vi "MR_Build-A-Block.vi"(1 "Build-A-Block":T2(array[cluster])=[{"Row Type Selector"=enum."Wait (minutes)", "Index"=0.0, "Direction"=enum."Forward"}, {"Row Type Selector"=enum."Vertical Profile", "Index"=0.0, "Direction"=enum."Forward"}, {"Row Type Selector"=enum."Vertical Profile", "Index"=1.0, "Direction"=enum."Forward"}, {"Row Type Selector"=enum."Move Traverse Only", "Index"=0.0, "Direction"=enum."Forward"}, {"Row Type Selector"=enum."Send Message", "Index"=0.0, "Direction"=enum."Forward"}, {"Row Type Selector"=enum."Blank Row", "Index"=0.0, "Direction"=enum."Forward"}]) -> (0 "TaskArray":T5(array[cluster])=[{"Start X"=-3390.0, "Start Y"=-113.0, "Start Z"=780.0, "End X"=-3390.0, "End Y"=-113.0, "End Z"=780.0, "No. of pts."=0, "Spacing"=enum."Linear", "Filename"=path "", "Tunnel Speed"=7.64, "Averaging time (min)"=0.0, "Extra Commands"="", "Carrier_1 Q (l/min)"=0.0, "Carrier_2 Q (l/min)"=0.0, "Trace Gas Concentration (%)"=0.0, "Specific Arguments"="", "Comments"="Tunnel Warm Up", "Row No"=0, "Row Type Selector"=enum."Set Tunnel Speed Only", "Completion time"="", "Row Duration (mins)"=10.0, "No. of Valid pts."=0, "Meas Setup File"=""}, {"Start X"=-3390.0, "Start Y"=-113.0, "Start Z"=780.0, "End X"=-3390.0, "End Y"=-113.0, "End Z"=780.0, "No. of pts."=0, "Spacing"=enum."Linear", "Filename"=path "", "Tunnel Speed"=7.64, "Averaging time (min)"=0.0, "Extra Commands"="", "Carrier_1 Q (l/min)"=0.0, "Carrier_2 Q (l/min)"=0.0, "Trace Gas Concentration (%)"=0.0, "Specific Arguments"="10", "Comments"="Tunnel Warm Up", "Row No"=0, "Row Type Selector"=enum."Wait (minutes)", "Completion time"="", "Row Duration (mins)"=0.0, "No. of Valid pts."=0, "Meas Setup File"=""}, {"Start X"=0.0, "Start Y"=0.0, "Start Z"=150.0, "End X"=0.0, "End Y"=0.0, "End Z"=150.0, "No. of pts."=0, "Spacing"=enum."Linear", "Filename"=path "", "Tunnel Speed"=7.64, "Averaging time (min)"=0.0, "Extra Commands"="!Work in Tunnel Coordinates", "Carrier_1 Q (l/min)"=0.0, "Carrier_2 Q (l/min)"=0.0, "Trace Gas Concentration (%)"=0.0, "Specific Arguments"="", "Comments"="", "Row No"=0, "Row Type Selector"=enum."Move Traverse Only", "Completion time"="", "Row Duration (mins)"=0.0, "No. of Valid pts."=0, "Meas Setup File"=""}, {"Start X"=0.0, "Start Y"=0.0, "Start Z"=805.0, "End X"=0.0, "End Y"=0.0, "End Z"=805.0, "No. of pts."=0, "Spacing"=enum."Linear", "Filename"=path "", "Tunnel Speed"=7.64, "Averaging time (min)"=0.0, "Extra Commands"="!Work in Tunnel Coordinates", "Carrier_1 Q (l/min)"=0.0, "Carrier_2 Q (l/min)"=0.0, "Trace Gas Concentration (%)"=0.0, "Specific Arguments"="MoveTT.vi;10", "Comments"="", "Row No"=0, "Row Type Selector"=enum."Run VI Named:", "Completion time"="", "Row Duration (mins)"=0.0, "No. of Valid pts."=0, "Meas Setup File"=""}, {"Start X"=-72.9, "Start Y"=-56.5, "Start Z"=12.7, "End X"=-72.9, "End Y"=-56.5, "End Z"=25.4, "No. of pts."=3, "Spacing"=enum."Specified", "Filename"=path "M:/\\Projects\\8773\\Results\\Tunnel1\\AnemometerSurvey.xls", "Tunnel Speed"=7.64, "Averaging time (min)"=1.0, "Extra Commands"="", "Carrier_1 Q (l/min)"=0.0, "Carrier_2 Q (l/min)"=0.0, "Trace Gas Concentration (%)"=0.0, "Specific Arguments"="Z= ;12.7;19.1;25.4\r", "Comments"="Anemo1", "Row No"=0, "Row Type Selector"=enum."Vertical Profile", "Completion time"="", "Row Duration (mins)"=0.0, "No. of Valid pts."=0, "Meas Setup File"="Current_Setup.xls"}, {"Start X"=-458.4, "Start Y"=87.9, "Start Z"=25.6, "End X"=-458.4, "End Y"=87.9, "End Z"=38.3, "No. of pts."=3, "Spacing"=enum."Specified", "Filename"=path "M:/\\Projects\\8773\\Results\\Tunnel1\\AnemometerSurvey.xls", "Tunnel Speed"=7.64, "Averaging time (min)"=1.0, "Extra Commands"="", "Carrier_1 Q (l/min)"=0.0, "Carrier_2 Q (l/min)"=0.0, "Trace Gas Concentration (%)"=0.0, "Specific Arguments"="Z= ;25.6;32.0;38.3\r", "Comments"="Anemo2", "Row No"=0, "Row Type Selector"=enum."Vertical Profile", "Completion time"="", "Row Duration (mins)"=0.0, "No. of Valid pts."=0, "Meas Setup File"="Current_Setup.xls"}, {"Start X"=0.0, "Start Y"=0.0, "Start Z"=150.0, "End X"=0.0, "End Y"=0.0, "End Z"=150.0, "No. of pts."=0, "Spacing"=enum."Linear", "Filename"=path "", "Tunnel Speed"=7.64, "Averaging time (min)"=0.0, "Extra Commands"="!Work in Tunnel Coordinates", "Carrier_1 Q (l/min)"=0.0, "Carrier_2 Q (l/min)"=0.0, "Trace Gas Concentration (%)"=0.0, "Specific Arguments"="", "Comments"="", "Row No"=0, "Row Type Selector"=enum."Move Traverse Only", "Completion time"="", "Row Duration (mins)"=0.0, "No. of Valid pts."=0, "Meas Setup File"=""}, {"Start X"=0.0, "Start Y"=0.0, "Start Z"=805.0, "End X"=0.0, "End Y"=0.0, "End Z"=805.0, "No. of pts."=0, "Spacing"=enum."Linear", "Filename"=path "", "Tunnel Speed"=7.64, "Averaging time (min)"=0.0, "Extra Commands"="!Work in Tunnel Coordinates", "Carrier_1 Q (l/min)"=0.0, "Carrier_2 Q (l/min)"=0.0, "Trace Gas Concentration (%)"=0.0, "Specific Arguments"="MoveTT.vi;30", "Comments"="", "Row No"=0, "Row Type Selector"=enum."Run VI Named:", "Completion time"="", "Row Duration (mins)"=0.0, "No. of Valid pts."=0, "Meas Setup File"=""}, {"Start X"=-72.9, "Start Y"=-56.5, "Start Z"=12.7, "End X"=-72.9, "End Y"=-56.5, "End Z"=25.4, "No. of pts."=3, "Spacing"=enum."Specified", "Filename"=path "M:/\\Projects\\8773\\Results\\Tunnel1\\AnemometerSurvey.xls", "Tunnel Speed"=7.64, "Averaging time (min)"=1.0, "Extra Commands"="", "Carrier_1 Q (l/min)"=0.0, "Carrier_2 Q (l/min)"=0.0, "Trace Gas Concentration (%)"=0.0, "Specific Arguments"="Z= ;12.7;19.1;25.4\r", "Comments"="Anemo1", "Row No"=0, "Row Type Selector"=enum."Vertical Profile", "Completion time"="", "Row Duration (mins)"=0.0, "No. of Valid pts."=0, "Meas Setup File"="Current_Setup.xls"}, {"Start X"=-458.4, "Start Y"=87.9, "Start Z"=25.6, "End X"=-458.4, "End Y"=87.9, "End Z"=38.3, "No. of pts."=3, "Spacing"=enum."Specified", "Filename"=path "M:/\\Projects\\8773\\Results\\Tunnel1\\AnemometerSurvey.xls", "Tunnel Speed"=7.64, "Averaging time (min)"=1.0, "Extra Commands"="", "Carrier_1 Q (l/min)"=0.0, "Carrier_2 Q (l/min)"=0.0, "Trace Gas Concentration (%)"=0.0, "Specific Arguments"="Z= ;25.6;32.0;38.3\r", "Comments"="Anemo2", "Row No"=0, "Row Type Selector"=enum."Vertical Profile", "Completion time"="", "Row Duration (mins)"=0.0, "No. of Valid pts."=0, "Meas Setup File"="Current_Setup.xls"}, {"Start X"=0.0, "Start Y"=0.0, "Start Z"=150.0, "End X"=0.0, "End Y"=0.0, "End Z"=150.0, "No. of pts."=0, "Spacing"=enum."Linear", "Filename"=path "", "Tunnel Speed"=7.64, "Averaging time (min)"=0.0, "Extra Commands"="!Work in Tunnel Coordinates", "Carrier_1 Q (l/min)"=0.0, "Carrier_2 Q (l/min)"=0.0, "Trace Gas Concentration (%)"=0.0, "Specific Arguments"="", "Comments"="", "Row No"=0, "Row Type Selector"=enum."Move Traverse Only", "Completion time"="", "Row Duration (mins)"=0.0, "No. of Valid pts."=0, "Meas Setup File"=""}, {"Start X"=0.0, "Start Y"=0.0, "Start Z"=805.0, "End X"=0.0, "End Y"=0.0, "End Z"=805.0, "No. of pts."=0, "Spacing"=enum."Linear", "Filename"=path "", "Tunnel Speed"=7.64, "Averaging time (min)"=0.0, "Extra Commands"="!Work in Tunnel Coordinates", "Carrier_1 Q (l/min)"=0.0, "Carrier_2 Q (l/min)"=0.0, "Trace Gas Concentration (%)"=0.0, "Specific Arguments"="MoveTT.vi;50", "Comments"="", "Row No"=0, "Row Type Selector"=enum."Run VI Named:", "Completion time"="", "Row Duration (mins)"=0.0, "No. of Valid pts."=0, "Meas Setup File"=""}, {"Start X"=-72.9, "Start Y"=-56.5, "Start Z"=12.7, "End X"=-72.9, "End Y"=-56.5, "End Z"=25.4, "No. of pts."=3, "Spacing"=enum."Specified", "Filename"=path "M:/\\Projects\\8773\\Results\\Tunnel1\\AnemometerSurvey.xls", "Tunnel Speed"=7.64, "Averaging time (min)"=1.0, "Extra Commands"="", "Carrier_1 Q (l/min)"=0.0, "Carrier_2 Q (l/min)"=0.0, "Trace Gas Concentration (%)"=0.0, "Specific Arguments"="Z= ;12.7;19.1;25.4\r", "Comments"="Anemo1", "Row No"=0, "Row Type Selector"=enum."Vertical Profile", "Completion time"="", "Row Duration (mins)"=0.0, "No. of Valid pts."=0, "Meas Setup File"="Current_Setup.xls"}, {"Start X"=-458.4, "Start Y"=87.9, "Start Z"=25.6, "End X"=-458.4, "End Y"=87.9, "End Z"=38.3, "No. of pts."=3, "Spacing"=enum."Specified", "Filename"=path "M:/\\Projects\\8773\\Results\\Tunnel1\\AnemometerSurvey.xls", "Tunnel Speed"=7.64, "Averaging time (min)"=1.0, "Extra Commands"="", "Carrier_1 Q (l/min)"=0.0, "Carrier_2 Q (l/min)"=0.0, "Trace Gas Concentration (%)"=0.0, "Specific Arguments"="Z= ;25.6;32.0;38.3\r", "Comments"="Anemo2", "Row No"=0, "Row Type Selector"=enum."Vertical Profile", "Completion time"="", "Row Duration (mins)"=0.0, "No. of Valid pts."=0, "Meas Setup File"="Current_Setup.xls"}, {"Start X"=0.0, "Start Y"=0.0, "Start Z"=150.0, "End X"=0.0, "End Y"=0.0, "End Z"=150.0, "No. of pts."=0, "Spacing"=enum."Linear", "Filename"=path "", "Tunnel Speed"=7.64, "Averaging time (min)"=0.0, "Extra Commands"="!Work in Tunnel Coordinates", "Carrier_1 Q (l/min)"=0.0, "Carrier_2 Q (l/min)"=0.0, "Trace Gas Concentration (%)"=0.0, "Specific Arguments"="", "Comments"="", "Row No"=0, "Row Type Selector"=enum."Move Traverse Only", "Completion time"="", "Row Duration (mins)"=0.0, "No. of Valid pts."=0, "Meas Setup File"=""}, {"Start X"=0.0, "Start Y"=0.0, "Start Z"=805.0, "End X"=0.0, "End Y"=0.0, "End Z"=805.0, "No. of pts."=0, "Spacing"=enum."Linear", "Filename"=path "", "Tunnel Speed"=7.64, "Averaging time (min)"=0.0, "Extra Commands"="!Work in Tunnel Coordinates", "Carrier_1 Q (l/min)"=0.0, "Carrier_2 Q (l/min)"=0.0, "Trace Gas Concentration (%)"=0.0, "Specific Arguments"="MoveTT.vi;70", "Comments"="", "Row No"=0, "Row Type Selector"=enum."Run VI Named:", "Completion time"="", "Row Duration (mins)"=0.0, "No. of Valid pts."=0, "Meas Setup File"=""}, {"Start X"=-72.9, "Start Y"=-56.5, "Start Z"=12.7, "End X"=-72.9, "End Y"=-56.5, "End Z"=25.4, "No. of pts."=3, "Spacing"=enum."Specified", "Filename"=path "M:/\\Projects\\8773\\Results\\Tunnel1\\AnemometerSurvey.xls", "Tunnel Speed"=7.64, "Averaging time (min)"=1.0, "Extra Commands"="", "Carrier_1 Q (l/min)"=0.0, "Carrier_2 Q (l/min)"=0.0, "Trace Gas Concentration (%)"=0.0, "Specific Arguments"="Z= ;12.7;19.1;25.4\r", "Comments"="Anemo1", "Row No"=0, "Row Type Selector"=enum."Vertical Profile", "Completion time"="", "Row Duration (mins)"=0.0, "No. of Valid pts."=0, "Meas Setup File"="Current_Setup.xls"}, {"Start X"=-458.4, "Start Y"=87.9, "Start Z"=25.6, "End X"=-458.4, "End Y"=87.9, "End Z"=38.3, "No. of pts."=3, "Spacing"=enum."Specified", "Filename"=path "M:/\\Projects\\8773\\Results\\Tunnel1\\AnemometerSurvey.xls", "Tunnel Speed"=7.64, "Averaging time (min)"=1.0, "Extra Commands"="", "Carrier_1 Q (l/min)"=0.0, "Carrier_2 Q (l/min)"=0.0, "Trace Gas Concentration (%)"=0.0, "Specific Arguments"="Z= ;25.6;32.0;38.3\r", "Comments"="Anemo2", "Row No"=0, "Row Type Selector"=enum."Vertical Profile", "Completion time"="", "Row Duration (mins)"=0.0, "No. of Valid pts."=0, "Meas Setup File"="Current_Setup.xls"}, {"Start X"=0.0, "Start Y"=0.0, "Start Z"=150.0, "End X"=0.0, "End Y"=0.0, "End Z"=150.0, "No. of pts."=0, "Spacing"=enum."Linear", "Filename"=path "", "Tunnel Speed"=7.64, "Averaging time (min)"=0.0, "Extra Commands"="!Work in Tunnel Coordinates", "Carrier_1 Q (l/min)"=0.0, "Carrier_2 Q (l/min)"=0.0, "Trace Gas Concentration (%)"=0.0, "Specific Arguments"="", "Comments"="", "Row No"=0, "Row Type Selector"=enum."Move Traverse Only", "Completion time"="", "Row Duration (mins)"=0.0, "No. of Valid pts."=0, "Meas Setup File"=""}, {"Start X"=0.0, "Start Y"=0.0, "Start Z"=805.0, "End X"=0.0, "End Y"=0.0, "End Z"=805.0, "No. of pts."=0, "Spacing"=enum."Linear", "Filename"=path "", "Tunnel Speed"=7.64, "Averaging time (min)"=0.0, "Extra Commands"="!Work in Tunnel Coordinates", "Carrier_1 Q (l/min)"=0.0, "Carrier_2 Q (l/min)"=0.0, "Trace Gas Concentration (%)"=0.0, "Specific Arguments"="MoveTT.vi;90", "Comments"="", "Row No"=0, "Row Type Selector"=enum."Run VI Named:", "Completion time"="", "Row Duration (mins)"=0.0, "No. of Valid pts."=0, "Meas Setup File"=""}, {"Start X"=-72.9, "Start Y"=-56.5, "Start Z"=12.7, "End X"=-72.9, "End Y"=-56.5, "End Z"=25.4, "No. of pts."=3, "Spacing"=enum."Specified", "Filename"=path "M:/\\Projects\\8773\\Results\\Tunnel1\\AnemometerSurvey.xls", "Tunnel Speed"=7.64, "Averaging time (min)"=1.0, "Extra Commands"="", "Carrier_1 Q (l/min)"=0.0, "Carrier_2 Q (l/min)"=0.0, "Trace Gas Concentration (%)"=0.0, "Specific Arguments"="Z= ;12.7;19.1;25.4\r", "Comments"="Anemo1", "Row No"=0, "Row Type Selector"=enum."Vertical Profile", "Completion time"="", "Row Duration (mins)"=0.0, "No. of Valid pts."=0, "Meas Setup File"="Current_Setup.xls"}, {"Start X"=-458.4, "Start Y"=87.9, "Start Z"=25.6, "End X"=-458.4, "End Y"=87.9, "End Z"=38.3, "No. of pts."=3, "Spacing"=enum."Specified", "Filename"=path "M:/\\Projects\\8773\\Results\\Tunnel1\\AnemometerSurvey.xls", "Tunnel Speed"=7.64, "Averaging time (min)"=1.0, "Extra Commands"="", "Carrier_1 Q (l/min)"=0.0, "Carrier_2 Q (l/min)"=0.0, "Trace Gas Concentration (%)"=0.0, "Specific Arguments"="Z= ;25.6;32.0;38.3\r", "Comments"="Anemo2", "Row No"=0, "Row Type Selector"=enum."Vertical Profile", "Completion time"="", "Row Duration (mins)"=0.0, "No. of Valid pts."=0, "Meas Setup File"="Current_Setup.xls"}, {"Start X"=0.0, "Start Y"=0.0, "Start Z"=150.0, "End X"=0.0, "End Y"=0.0, "End Z"=150.0, "No. of pts."=0, "Spacing"=enum."Linear", "Filename"=path "", "Tunnel Speed"=7.64, "Averaging time (min)"=0.0, "Extra Commands"="!Work in Tunnel Coordinates", "Carrier_1 Q (l/min)"=0.0, "Carrier_2 Q (l/min)"=0.0, "Trace Gas Concentration (%)"=0.0, "Specific Arguments"="", "Comments"="", "Row No"=0, "Row Type Selector"=enum."Move Traverse Only", "Completion time"="", "Row Duration (mins)"=0.0, "No. of Valid pts."=0, "Meas Setup File"=""}, {"Start X"=0.0, "Start Y"=0.0, "Start Z"=805.0, "End X"=0.0, "End Y"=0.0, "End Z"=805.0, "No. of pts."=0, "Spacing"=enum."Linear", "Filename"=path "", "Tunnel Speed"=7.64, "Averaging time (min)"=0.0, "Extra Commands"="!Work in Tunnel Coordinates", "Carrier_1 Q (l/min)"=0.0, "Carrier_2 Q (l/min)"=0.0, "Trace Gas Concentration (%)"=0.0, "Specific Arguments"="MoveTT.vi;110", "Comments"="", "Row No"=0, "Row Type Selector"=enum."Run VI Named:", "Completion time"="", "Row Duration (mins)"=0.0, "No. of Valid pts."=0, "Meas Setup File"=""}, {"Start X"=-72.9, "Start Y"=-56.5, "Start Z"=12.7, "End X"=-72.9, "End Y"=-56.5, "End Z"=25.4, "No. of pts."=3, "Spacing"=enum."Specified", "Filename"=path "M:/\\Projects\\8773\\Results\\Tunnel1\\AnemometerSurvey.xls", "Tunnel Speed"=7.64, "Averaging time (min)"=1.0, "Extra Commands"="", "Carrier_1 Q (l/min)"=0.0, "Carrier_2 Q (l/min)"=0.0, "Trace Gas Concentration (%)"=0.0, "Specific Arguments"="Z= ;12.7;19.1;25.4\r", "Comments"="Anemo1", "Row No"=0, "Row Type Selector"=enum."Vertical Profile", "Completion time"="", "Row Duration (mins)"=0.0, "No. of Valid pts."=0, "Meas Setup File"="Current_Setup.xls"}, {"Start X"=-458.4, "Start Y"=87.9, "Start Z"=25.6, "End X"=-458.4, "End Y"=87.9, "End Z"=38.3, "No. of pts."=3, "Spacing"=enum."Specified", "Filename"=path "M:/\\Projects\\8773\\Results\\Tunnel1\\AnemometerSurvey.xls", "Tunnel Speed"=7.64, "Averaging time (min)"=1.0, "Extra Commands"="", "Carrier_1 Q (l/min)"=0.0, "Carrier_2 Q (l/min)"=0.0, "Trace Gas Concentration (%)"=0.0, "Specific Arguments"="Z= ;25.6;32.0;38.3\r", "Comments"="Anemo2", "Row No"=0, "Row Type Selector"=enum."Vertical Profile", "Completion time"="", "Row Duration (mins)"=0.0, "No. of Valid pts."=0, "Meas Setup File"="Current_Setup.xls"}, {"Start X"=0.0, "Start Y"=0.0, "Start Z"=150.0, "End X"=0.0, "End Y"=0.0, "End Z"=150.0, "No. of pts."=0, "Spacing"=enum."Linear", "Filename"=path "", "Tunnel Speed"=7.64, "Averaging time (min)"=0.0, "Extra Commands"="!Work in Tunnel Coordinates", "Carrier_1 Q (l/min)"=0.0, "Carrier_2 Q (l/min)"=0.0, "Trace Gas Concentration (%)"=0.0, "Specific Arguments"="", "Comments"="", "Row No"=0, "Row Type Selector"=enum."Move Traverse Only", "Completion time"="", "Row Duration (mins)"=0.0, "No. of Valid pts."=0, "Meas Setup File"=""}, {"Start X"=0.0, "Start Y"=0.0, "Start Z"=805.0, "End X"=0.0, "End Y"=0.0, "End Z"=805.0, "No. of pts."=0, "Spacing"=enum."Linear", "Filename"=path "", "Tunnel Speed"=7.64, "Averaging time (min)"=0.0, "Extra Commands"="!Work in Tunnel Coordinates", "Carrier_1 Q (l/min)"=0.0, "Carrier_2 Q (l/min)"=0.0, "Trace Gas Concentration (%)"=0.0, "Specific Arguments"="MoveTT.vi;130", "Comments"="", "Row No"=0, "Row Type Selector"=enum."Run VI Named:", "Completion time"="", "Row Duration (mins)"=0.0, "No. of Valid pts."=0, "Meas Setup File"=""}, {"Start X"=-72.9, "Start Y"=-56.5, "Start Z"=12.7, "End X"=-72.9, "End Y"=-56.5, "End Z"=25.4, "No. of pts."=3, "Spacing"=enum."Specified", "Filename"=path "M:/\\Projects\\8773\\Results\\Tunnel1\\AnemometerSurvey.xls", "Tunnel Speed"=7.64, "Averaging time (min)"=1.0, "Extra Commands"="", "Carrier_1 Q (l/min)"=0.0, "Carrier_2 Q (l/min)"=0.0, "Trace Gas Concentration (%)"=0.0, "Specific Arguments"="Z= ;12.7;19.1;25.4\r", "Comments"="Anemo1", "Row No"=0, "Row Type Selector"=enum."Vertical Profile", "Completion time"="", "Row Duration (mins)"=0.0, "No. of Valid pts."=0, "Meas Setup File"="Current_Setup.xls"}, {"Start X"=-458.4, "Start Y"=87.9, "Start Z"=25.6, "End X"=-458.4, "End Y"=87.9, "End Z"=38.3, "No. of pts."=3, "Spacing"=enum."Specified", "Filename"=path "M:/\\Projects\\8773\\Results\\Tunnel1\\AnemometerSurvey.xls", "Tunnel Speed"=7.64, "Averaging time (min)"=1.0, "Extra Commands"="", "Carrier_1 Q (l/min)"=0.0, "Carrier_2 Q (l/min)"=0.0, "Trace Gas Concentration (%)"=0.0, "Specific Arguments"="Z= ;25.6;32.0;38.3\r", "Comments"="Anemo2", "Row No"=0, "Row Type Selector"=enum."Vertical Profile", "Completion time"="", "Row Duration (mins)"=0.0, "No. of Valid pts."=0, "Meas Setup File"="Current_Setup.xls"}, {"Start X"=0.0, "Start Y"=0.0, "Start Z"=150.0, "End X"=0.0, "End Y"=0.0, "End Z"=150.0, "No. of pts."=0, "Spacing"=enum."Linear", "Filename"=path "", "Tunnel Speed"=7.64, "Averaging time (min)"=0.0, "Extra Commands"="!Work in Tunnel Coordinates", "Carrier_1 Q (l/min)"=0.0, "Carrier_2 Q (l/min)"=0.0, "Trace Gas Concentration (%)"=0.0, "Specific Arguments"="", "Comments"="", "Row No"=0, "Row Type Selector"=enum."Move Traverse Only", "Completion time"="", "Row Duration (mins)"=0.0, "No. of Valid pts."=0, "Meas Setup File"=""}, {"Start X"=0.0, "Start Y"=0.0, "Start Z"=805.0, "End X"=0.0, "End Y"=0.0, "End Z"=805.0, "No. of pts."=0, "Spacing"=enum."Linear", "Filename"=path "", "Tunnel Speed"=7.64, "Averaging time (min)"=0.0, "Extra Commands"="!Work in Tunnel Coordinates", "Carrier_1 Q (l/min)"=0.0, "Carrier_2 Q (l/min)"=0.0, "Trace Gas Concentration (%)"=0.0, "Specific Arguments"="MoveTT.vi;150", "Comments"="", "Row No"=0, "Row Type Selector"=enum."Run VI Named:", "Completion time"="", "Row Duration (mins)"=0.0, "No. of Valid pts."=0, "Meas Setup File"=""}, {"Start X"=-72.9, "Start Y"=-56.5, "Start Z"=12.7, "End X"=-72.9, "End Y"=-56.5, "End Z"=25.4, "No. of pts."=3, "Spacing"=enum."Specified", "Filename"=path "M:/\\Projects\\8773\\Results\\Tunnel1\\AnemometerSurvey.xls", "Tunnel Speed"=7.64, "Averaging time (min)"=1.0, "Extra Commands"="", "Carrier_1 Q (l/min)"=0.0, "Carrier_2 Q (l/min)"=0.0, "Trace Gas Concentration (%)"=0.0, "Specific Arguments"="Z= ;12.7;19.1;25.4\r", "Comments"="Anemo1", "Row No"=0, "Row Type Selector"=enum."Vertical Profile", "Completion time"="", "Row Duration (mins)"=0.0, "No. of Valid pts."=0, "Meas Setup File"="Current_Setup.xls"}, {"Start X"=-458.4, "Start Y"=87.9, "Start Z"=25.6, "End X"=-458.4, "End Y"=87.9, "End Z"=38.3, "No. of pts."=3, "Spacing"=enum."Specified", "Filename"=path "M:/\\Projects\\8773\\Results\\Tunnel1\\AnemometerSurvey.xls", "Tunnel Speed"=7.64, "Averaging time (min)"=1.0, "Extra Commands"="", "Carrier_1 Q (l/min)"=0.0, "Carrier_2 Q (l/min)"=0.0, "Trace Gas Concentration (%)"=0.0, "Specific Arguments"="Z= ;25.6;32.0;38.3\r", "Comments"="Anemo2", "Row No"=0, "Row Type Selector"=enum."Vertical Profile", "Completion time"="", "Row Duration (mins)"=0.0, "No. of Valid pts."=0, "Meas Setup File"="Current_Setup.xls"}, {"Start X"=0.0, "Start Y"=0.0, "Start Z"=150.0, "End X"=0.0, "End Y"=0.0, "End Z"=150.0, "No. of pts."=0, "Spacing"=enum."Linear", "Filename"=path "", "Tunnel Speed"=7.64, "Averaging time (min)"=0.0, "Extra Commands"="!Work in Tunnel Coordinates", "Carrier_1 Q (l/min)"=0.0, "Carrier_2 Q (l/min)"=0.0, "Trace Gas Concentration (%)"=0.0, "Specific Arguments"="", "Comments"="", "Row No"=0, "Row Type Selector"=enum."Move Traverse Only", "Completion time"="", "Row Duration (mins)"=0.0, "No. of Valid pts."=0, "Meas Setup File"=""}, {"Start X"=0.0, "Start Y"=0.0, "Start Z"=805.0, "End X"=0.0, "End Y"=0.0, "End Z"=805.0, "No. of pts."=0, "Spacing"=enum."Linear", "Filename"=path "", "Tunnel Speed"=7.64, "Averaging time (min)"=0.0, "Extra Commands"="!Work in Tunnel Coordinates", "Carrier_1 Q (l/min)"=0.0, "Carrier_2 Q (l/min)"=0.0, "Trace Gas Concentration (%)"=0.0, "Specific Arguments"="MoveTT.vi;170", "Comments"="", "Row No"=0, "Row Type Selector"=enum."Run VI Named:", "Completion time"="", "Row Duration (mins)"=0.0, "No. of Valid pts."=0, "Meas Setup File"=""}, {"Start X"=-72.9, "Start Y"=-56.5, "Start Z"=12.7, "End X"=-72.9, "End Y"=-56.5, "End Z"=25.4, "No. of pts."=3, "Spacing"=enum."Specified", "Filename"=path "M:/\\Projects\\8773\\Results\\Tunnel1\\AnemometerSurvey.xls", "Tunnel Speed"=7.64, "Averaging time (min)"=1.0, "Extra Commands"="", "Carrier_1 Q (l/min)"=0.0, "Carrier_2 Q (l/min)"=0.0, "Trace Gas Concentration (%)"=0.0, "Specific Arguments"="Z= ;12.7;19.1;25.4\r", "Comments"="Anemo1", "Row No"=0, "Row Type Selector"=enum."Vertical Profile", "Completion time"="", "Row Duration (mins)"=0.0, "No. of Valid pts."=0, "Meas Setup File"="Current_Setup.xls"}, {"Start X"=-458.4, "Start Y"=87.9, "Start Z"=25.6, "End X"=-458.4, "End Y"=87.9, "End Z"=38.3, "No. of pts."=3, "Spacing"=enum."Specified", "Filename"=path "M:/\\Projects\\8773\\Results\\Tunnel1\\AnemometerSurvey.xls", "Tunnel Speed"=7.64, "Averaging time (min)"=1.0, "Extra Commands"="", "Carrier_1 Q (l/min)"=0.0, "Carrier_2 Q (l/min)"=0.0, "Trace Gas Concentration (%)"=0.0, "Specific Arguments"="Z= ;25.6;32.0;38.3\r", "Comments"="Anemo2", "Row No"=0, "Row Type Selector"=enum."Vertical Profile", "Completion time"="", "Row Duration (mins)"=0.0, "No. of Valid pts."=0, "Meas Setup File"="Current_Setup.xls"}, {"Start X"=0.0, "Start Y"=0.0, "Start Z"=150.0, "End X"=0.0, "End Y"=0.0, "End Z"=150.0, "No. of pts."=0, "Spacing"=enum."Linear", "Filename"=path "", "Tunnel Speed"=7.64, "Averaging time (min)"=0.0, "Extra Commands"="!Work in Tunnel Coordinates", "Carrier_1 Q (l/min)"=0.0, "Carrier_2 Q (l/min)"=0.0, "Trace Gas Concentration (%)"=0.0, "Specific Arguments"="", "Comments"="", "Row No"=0, "Row Type Selector"=enum."Move Traverse Only", "Completion time"="", "Row Duration (mins)"=0.0, "No. of Valid pts."=0, "Meas Setup File"=""}, {"Start X"=0.0, "Start Y"=0.0, "Start Z"=805.0, "End X"=0.0, "End Y"=0.0, "End Z"=805.0, "No. of pts."=0, "Spacing"=enum."Linear", "Filename"=path "", "Tunnel Speed"=7.64, "Averaging time (min)"=0.0, "Extra Commands"="!Work in Tunnel Coordinates", "Carrier_1 Q (l/min)"=0.0, "Carrier_2 Q (l/min)"=0.0, "Trace Gas Concentration (%)"=0.0, "Specific Arguments"="MoveTT.vi;190", "Comments"="", "Row No"=0, "Row Type Selector"=enum."Run VI Named:", "Completion time"="", "Row Duration (mins)"=0.0, "No. of Valid pts."=0, "Meas Setup File"=""}, {"Start X"=-72.9, "Start Y"=-56.5, "Start Z"=12.7, "End X"=-72.9, "End Y"=-56.5, "End Z"=25.4, "No. of pts."=3, "Spacing"=enum."Specified", "Filename"=path "M:/\\Projects\\8773\\Results\\Tunnel1\\AnemometerSurvey.xls", "Tunnel Speed"=7.64, "Averaging time (min)"=1.0, "Extra Commands"="", "Carrier_1 Q (l/min)"=0.0, "Carrier_2 Q (l/min)"=0.0, "Trace Gas Concentration (%)"=0.0, "Specific Arguments"="Z= ;12.7;19.1;25.4\r", "Comments"="Anemo1", "Row No"=0, "Row Type Selector"=enum."Vertical Profile", "Completion time"="", "Row Duration (mins)"=0.0, "No. of Valid pts."=0, "Meas Setup File"="Current_Setup.xls"}, {"Start X"=-458.4, "Start Y"=87.9, "Start Z"=25.6, "End X"=-458.4, "End Y"=87.9, "End Z"=38.3, "No. of pts."=3, "Spacing"=enum."Specified", "Filename"=path "M:/\\Projects\\8773\\Results\\Tunnel1\\AnemometerSurvey.xls", "Tunnel Speed"=7.64, "Averaging time (min)"=1.0, "Extra Commands"="", "Carrier_1 Q (l/min)"=0.0, "Carrier_2 Q (l/min)"=0.0, "Trace Gas Concentration (%)"=0.0, "Specific Arguments"="Z= ;25.6;32.0;38.3\r", "Comments"="Anemo2", "Row No"=0, "Row Type Selector"=enum."Vertical Profile", "Completion time"="", "Row Duration (mins)"=0.0, "No. of Valid pts."=0, "Meas Setup File"="Current_Setup.xls"}, {"Start X"=0.0, "Start Y"=0.0, "Start Z"=150.0, "End X"=0.0, "End Y"=0.0, "End Z"=150.0, "No. of pts."=0, "Spacing"=enum."Linear", "Filename"=path "", "Tunnel Speed"=7.64, "Averaging time (min)"=0.0, "Extra Commands"="!Work in Tunnel Coordinates", "Carrier_1 Q (l/min)"=0.0, "Carrier_2 Q (l/min)"=0.0, "Trace Gas Concentration (%)"=0.0, "Specific Arguments"="", "Comments"="", "Row No"=0, "Row Type Selector"=enum."Move Traverse Only", "Completion time"="", "Row Duration (mins)"=0.0, "No. of Valid pts."=0, "Meas Setup File"=""}, {"Start X"=0.0, "Start Y"=0.0, "Start Z"=805.0, "End X"=0.0, "End Y"=0.0, "End Z"=805.0, "No. of pts."=0, "Spacing"=enum."Linear", "Filename"=path "", "Tunnel Speed"=7.64, "Averaging time (min)"=0.0, "Extra Commands"="!Work in Tunnel Coordinates", "Carrier_1 Q (l/min)"=0.0, "Carrier_2 Q (l/min)"=0.0, "Trace Gas Concentration (%)"=0.0, "Specific Arguments"="MoveTT.vi;210", "Comments"="", "Row No"=0, "Row Type Selector"=enum."Run VI Named:", "Completion time"="", "Row Duration (mins)"=0.0, "No. of Valid pts."=0, "Meas Setup File"=""}, {"Start X"=-72.9, "Start Y"=-56.5, "Start Z"=12.7, "End X"=-72.9, "End Y"=-56.5, "End Z"=25.4, "No. of pts."=3, "Spacing"=enum."Specified", "Filename"=path "M:/\\Projects\\8773\\Results\\Tunnel1\\AnemometerSurvey.xls", "Tunnel Speed"=7.64, "Averaging time (min)"=1.0, "Extra Commands"="", "Carrier_1 Q (l/min)"=0.0, "Carrier_2 Q (l/min)"=0.0, "Trace Gas Concentration (%)"=0.0, "Specific Arguments"="Z= ;12.7;19.1;25.4\r", "Comments"="Anemo1", "Row No"=0, "Row Type Selector"=enum."Vertical Profile", "Completion time"="", "Row Duration (mins)"=0.0, "No. of Valid pts."=0, "Meas Setup File"="Current_Setup.xls"}, {"Start X"=-458.4, "Start Y"=87.9, "Start Z"=25.6, "End X"=-458.4, "End Y"=87.9, "End Z"=38.3, "No. of pts."=3, "Spacing"=enum."Specified", "Filename"=path "M:/\\Projects\\8773\\Results\\Tunnel1\\AnemometerSurvey.xls", "Tunnel Speed"=7.64, "Averaging time (min)"=1.0, "Extra Commands"="", "Carrier_1 Q (l/min)"=0.0, "Carrier_2 Q (l/min)"=0.0, "Trace Gas Concentration (%)"=0.0, "Specific Arguments"="Z= ;25.6;32.0;38.3\r", "Comments"="Anemo2", "Row No"=0, "Row Type Selector"=enum."Vertical Profile", "Completion time"="", "Row Duration (mins)"=0.0, "No. of Valid pts."=0, "Meas Setup File"="Current_Setup.xls"}, {"Start X"=0.0, "Start Y"=0.0, "Start Z"=150.0, "End X"=0.0, "End Y"=0.0, "End Z"=150.0, "No. of pts."=0, "Spacing"=enum."Linear", "Filename"=path "", "Tunnel Speed"=7.64, "Averaging time (min)"=0.0, "Extra Commands"="!Work in Tunnel Coordinates", "Carrier_1 Q (l/min)"=0.0, "Carrier_2 Q (l/min)"=0.0, "Trace Gas Concentration (%)"=0.0, "Specific Arguments"="", "Comments"="", "Row No"=0, "Row Type Selector"=enum."Move Traverse Only", "Completion time"="", "Row Duration (mins)"=0.0, "No. of Valid pts."=0, "Meas Setup File"=""}, {"Start X"=0.0, "Start Y"=0.0, "Start Z"=805.0, "End X"=0.0, "End Y"=0.0, "End Z"=805.0, "No. of pts."=0, "Spacing"=enum."Linear", "Filename"=path "", "Tunnel Speed"=7.64, "Averaging time (min)"=0.0, "Extra Commands"="!Work in Tunnel Coordinates", "Carrier_1 Q (l/min)"=0.0, "Carrier_2 Q (l/min)"=0.0, "Trace Gas Concentration (%)"=0.0, "Specific Arguments"="MoveTT.vi;230", "Comments"="", "Row No"=0, "Row Type Selector"=enum."Run VI Named:", "Completion time"="", "Row Duration (mins)"=0.0, "No. of Valid pts."=0, "Meas Setup File"=""}, {"Start X"=-72.9, "Start Y"=-56.5, "Start Z"=12.7, "End X"=-72.9, "End Y"=-56.5, "End Z"=25.4, "No. of pts."=3, "Spacing"=enum."Specified", "Filename"=path "M:/\\Projects\\8773\\Results\\Tunnel1\\AnemometerSurvey.xls", "Tunnel Speed"=7.64, "Averaging time (min)"=1.0, "Extra Commands"="", "Carrier_1 Q (l/min)"=0.0, "Carrier_2 Q (l/min)"=0.0, "Trace Gas Concentration (%)"=0.0, "Specific Arguments"="Z= ;12.7;19.1;25.4\r", "Comments"="Anemo1", "Row No"=0, "Row Type Selector"=enum."Vertical Profile", "Completion time"="", "Row Duration (mins)"=0.0, "No. of Valid pts."=0, "Meas Setup File"="Current_Setup.xls"}, {"Start X"=-458.4, "Start Y"=87.9, "Start Z"=25.6, "End X"=-458.4, "End Y"=87.9, "End Z"=38.3, "No. of pts."=3, "Spacing"=enum."Specified", "Filename"=path "M:/\\Projects\\8773\\Results\\Tunnel1\\AnemometerSurvey.xls", "Tunnel Speed"=7.64, "Averaging time (min)"=1.0, "Extra Commands"="", "Carrier_1 Q (l/min)"=0.0, "Carrier_2 Q (l/min)"=0.0, "Trace Gas Concentration (%)"=0.0, "Specific Arguments"="Z= ;25.6;32.0;38.3\r", "Comments"="Anemo2", "Row No"=0, "Row Type Selector"=enum."Vertical Profile", "Completion time"="", "Row Duration (mins)"=0.0, "No. of Valid pts."=0, "Meas Setup File"="Current_Setup.xls"}, {"Start X"=0.0, "Start Y"=0.0, "Start Z"=150.0, "End X"=0.0, "End Y"=0.0, "End Z"=150.0, "No. of pts."=0, "Spacing"=enum."Linear", "Filename"=path "", "Tunnel Speed"=7.64, "Averaging time (min)"=0.0, "Extra Commands"="!Work in Tunnel Coordinates", "Carrier_1 Q (l/min)"=0.0, "Carrier_2 Q (l/min)"=0.0, "Trace Gas Concentration (%)"=0.0, "Specific Arguments"="", "Comments"="", "Row No"=0, "Row Type Selector"=enum."Move Traverse Only", "Completion time"="", "Row Duration (mins)"=0.0, "No. of Valid pts."=0, "Meas Setup File"=""}, {"Start X"=0.0, "Start Y"=0.0, "Start Z"=805.0, "End X"=0.0, "End Y"=0.0, "End Z"=805.0, "No. of pts."=0, "Spacing"=enum."Linear", "Filename"=path "", "Tunnel Speed"=7.64, "Averaging time (min)"=0.0, "Extra Commands"="!Work in Tunnel Coordinates", "Carrier_1 Q (l/min)"=0.0, "Carrier_2 Q (l/min)"=0.0, "Trace Gas Concentration (%)"=0.0, "Specific Arguments"="MoveTT.vi;250", "Comments"="", "Row No"=0, "Row Type Selector"=enum."Run VI Named:", "Completion time"="", "Row Duration (mins)"=0.0, "No. of Valid pts."=0, "Meas Setup File"=""}, {"Start X"=-72.9, "Start Y"=-56.5, "Start Z"=12.7, "End X"=-72.9, "End Y"=-56.5, "End Z"=25.4, "No. of pts."=3, "Spacing"=enum."Specified", "Filename"=path "M:/\\Projects\\8773\\Results\\Tunnel1\\AnemometerSurvey.xls", "Tunnel Speed"=7.64, "Averaging time (min)"=1.0, "Extra Commands"="", "Carrier_1 Q (l/min)"=0.0, "Carrier_2 Q (l/min)"=0.0, "Trace Gas Concentration (%)"=0.0, "Specific Arguments"="Z= ;12.7;19.1;25.4\r", "Comments"="Anemo1", "Row No"=0, "Row Type Selector"=enum."Vertical Profile", "Completion time"="", "Row Duration (mins)"=0.0, "No. of Valid pts."=0, "Meas Setup File"="Current_Setup.xls"}, {"Start X"=-458.4, "Start Y"=87.9, "Start Z"=25.6, "End X"=-458.4, "End Y"=87.9, "End Z"=38.3, "No. of pts."=3, "Spacing"=enum."Specified", "Filename"=path "M:/\\Projects\\8773\\Results\\Tunnel1\\AnemometerSurvey.xls", "Tunnel Speed"=7.64, "Averaging time (min)"=1.0, "Extra Commands"="", "Carrier_1 Q (l/min)"=0.0, "Carrier_2 Q (l/min)"=0.0, "Trace Gas Concentration (%)"=0.0, "Specific Arguments"="Z= ;25.6;32.0;38.3\r", "Comments"="Anemo2", "Row No"=0, "Row Type Selector"=enum."Vertical Profile", "Completion time"="", "Row Duration (mins)"=0.0, "No. of Valid pts."=0, "Meas Setup File"="Current_Setup.xls"}, {"Start X"=0.0, "Start Y"=0.0, "Start Z"=150.0, "End X"=0.0, "End Y"=0.0, "End Z"=150.0, "No. of pts."=0, "Spacing"=enum."Linear", "Filename"=path "", "Tunnel Speed"=7.64, "Averaging time (min)"=0.0, "Extra Commands"="!Work in Tunnel Coordinates", "Carrier_1 Q (l/min)"=0.0, "Carrier_2 Q (l/min)"=0.0, "Trace Gas Concentration (%)"=0.0, "Specific Arguments"="", "Comments"="", "Row No"=0, "Row Type Selector"=enum."Move Traverse Only", "Completion time"="", "Row Duration (mins)"=0.0, "No. of Valid pts."=0, "Meas Setup File"=""}, {"Start X"=0.0, "Start Y"=0.0, "Start Z"=805.0, "End X"=0.0, "End Y"=0.0, "End Z"=805.0, "No. of pts."=0, "Spacing"=enum."Linear", "Filename"=path "", "Tunnel Speed"=7.64, "Averaging time (min)"=0.0, "Extra Commands"="!Work in Tunnel Coordinates", "Carrier_1 Q (l/min)"=0.0, "Carrier_2 Q (l/min)"=0.0, "Trace Gas Concentration (%)"=0.0, "Specific Arguments"="MoveTT.vi;270", "Comments"="", "Row No"=0, "Row Type Selector"=enum."Run VI Named:", "Completion time"="", "Row Duration (mins)"=0.0, "No. of Valid pts."=0, "Meas Setup File"=""}, {"Start X"=-72.9, "Start Y"=-56.5, "Start Z"=12.7, "End X"=-72.9, "End Y"=-56.5, "End Z"=25.4, "No. of pts."=3, "Spacing"=enum."Specified", "Filename"=path "M:/\\Projects\\8773\\Results\\Tunnel1\\AnemometerSurvey.xls", "Tunnel Speed"=7.64, "Averaging time (min)"=1.0, "Extra Commands"="", "Carrier_1 Q (l/min)"=0.0, "Carrier_2 Q (l/min)"=0.0, "Trace Gas Concentration (%)"=0.0, "Specific Arguments"="Z= ;12.7;19.1;25.4\r", "Comments"="Anemo1", "Row No"=0, "Row Type Selector"=enum."Vertical Profile", "Completion time"="", "Row Duration (mins)"=0.0, "No. of Valid pts."=0, "Meas Setup File"="Current_Setup.xls"}, {"Start X"=-458.4, "Start Y"=87.9, "Start Z"=25.6, "End X"=-458.4, "End Y"=87.9, "End Z"=38.3, "No. of pts."=3, "Spacing"=enum."Specified", "Filename"=path "M:/\\Projects\\8773\\Results\\Tunnel1\\AnemometerSurvey.xls", "Tunnel Speed"=7.64, "Averaging time (min)"=1.0, "Extra Commands"="", "Carrier_1 Q (l/min)"=0.0, "Carrier_2 Q (l/min)"=0.0, "Trace Gas Concentration (%)"=0.0, "Specific Arguments"="Z= ;25.6;32.0;38.3\r", "Comments"="Anemo2", "Row No"=0, "Row Type Selector"=enum."Vertical Profile", "Completion time"="", "Row Duration (mins)"=0.0, "No. of Valid pts."=0, "Meas Setup File"="Current_Setup.xls"}, {"Start X"=0.0, "Start Y"=0.0, "Start Z"=150.0, "End X"=0.0, "End Y"=0.0, "End Z"=150.0, "No. of pts."=0, "Spacing"=enum."Linear", "Filename"=path "", "Tunnel Speed"=7.64, "Averaging time (min)"=0.0, "Extra Commands"="!Work in Tunnel Coordinates", "Carrier_1 Q (l/min)"=0.0, "Carrier_2 Q (l/min)"=0.0, "Trace Gas Concentration (%)"=0.0, "Specific Arguments"="", "Comments"="", "Row No"=0, "Row Type Selector"=enum."Move Traverse Only", "Completion time"="", "Row Duration (mins)"=0.0, "No. of Valid pts."=0, "Meas Setup File"=""}, {"Start X"=0.0, "Start Y"=0.0, "Start Z"=805.0, "End X"=0.0, "End Y"=0.0, "End Z"=805.0, "No. of pts."=0, "Spacing"=enum."Linear", "Filename"=path "", "Tunnel Speed"=7.64, "Averaging time (min)"=0.0, "Extra Commands"="!Work in Tunnel Coordinates", "Carrier_1 Q (l/min)"=0.0, "Carrier_2 Q (l/min)"=0.0, "Trace Gas Concentration (%)"=0.0, "Specific Arguments"="MoveTT.vi;290", "Comments"="", "Row No"=0, "Row Type Selector"=enum."Run VI Named:", "Completion time"="", "Row Duration (mins)"=0.0, "No. of Valid pts."=0, "Meas Setup File"=""}, {"Start X"=-72.9, "Start Y"=-56.5, "Start Z"=12.7, "End X"=-72.9, "End Y"=-56.5, "End Z"=25.4, "No. of pts."=3, "Spacing"=enum."Specified", "Filename"=path "M:/\\Projects\\8773\\Results\\Tunnel1\\AnemometerSurvey.xls", "Tunnel Speed"=7.64, "Averaging time (min)"=1.0, "Extra Commands"="", "Carrier_1 Q (l/min)"=0.0, "Carrier_2 Q (l/min)"=0.0, "Trace Gas Concentration (%)"=0.0, "Specific Arguments"="Z= ;12.7;19.1;25.4\r", "Comments"="Anemo1", "Row No"=0, "Row Type Selector"=enum."Vertical Profile", "Completion time"="", "Row Duration (mins)"=0.0, "No. of Valid pts."=0, "Meas Setup File"="Current_Setup.xls"}, {"Start X"=-458.4, "Start Y"=87.9, "Start Z"=25.6, "End X"=-458.4, "End Y"=87.9, "End Z"=38.3, "No. of pts."=3, "Spacing"=enum."Specified", "Filename"=path "M:/\\Projects\\8773\\Results\\Tunnel1\\AnemometerSurvey.xls", "Tunnel Speed"=7.64, "Averaging time (min)"=1.0, "Extra Commands"="", "Carrier_1 Q (l/min)"=0.0, "Carrier_2 Q (l/min)"=0.0, "Trace Gas Concentration (%)"=0.0, "Specific Arguments"="Z= ;25.6;32.0;38.3\r", "Comments"="Anemo2", "Row No"=0, "Row Type Selector"=enum."Vertical Profile", "Completion time"="", "Row Duration (mins)"=0.0, "No. of Valid pts."=0, "Meas Setup File"="Current_Setup.xls"}, {"Start X"=0.0, "Start Y"=0.0, "Start Z"=150.0, "End X"=0.0, "End Y"=0.0, "End Z"=150.0, "No. of pts."=0, "Spacing"=enum."Linear", "Filename"=path "", "Tunnel Speed"=7.64, "Averaging time (min)"=0.0, "Extra Commands"="!Work in Tunnel Coordinates", "Carrier_1 Q (l/min)"=0.0, "Carrier_2 Q (l/min)"=0.0, "Trace Gas Concentration (%)"=0.0, "Specific Arguments"="", "Comments"="", "Row No"=0, "Row Type Selector"=enum."Move Traverse Only", "Completion time"="", "Row Duration (mins)"=0.0, "No. of Valid pts."=0, "Meas Setup File"=""}, {"Start X"=0.0, "Start Y"=0.0, "Start Z"=805.0, "End X"=0.0, "End Y"=0.0, "End Z"=805.0, "No. of pts."=0, "Spacing"=enum."Linear", "Filename"=path "", "Tunnel Speed"=7.64, "Averaging time (min)"=0.0, "Extra Commands"="!Work in Tunnel Coordinates", "Carrier_1 Q (l/min)"=0.0, "Carrier_2 Q (l/min)"=0.0, "Trace Gas Concentration (%)"=0.0, "Specific Arguments"="MoveTT.vi;310", "Comments"="", "Row No"=0, "Row Type Selector"=enum."Run VI Named:", "Completion time"="", "Row Duration (mins)"=0.0, "No. of Valid pts."=0, "Meas Setup File"=""}, {"Start X"=-72.9, "Start Y"=-56.5, "Start Z"=12.7, "End X"=-72.9, "End Y"=-56.5, "End Z"=25.4, "No. of pts."=3, "Spacing"=enum."Specified", "Filename"=path "M:/\\Projects\\8773\\Results\\Tunnel1\\AnemometerSurvey.xls", "Tunnel Speed"=7.64, "Averaging time (min)"=1.0, "Extra Commands"="", "Carrier_1 Q (l/min)"=0.0, "Carrier_2 Q (l/min)"=0.0, "Trace Gas Concentration (%)"=0.0, "Specific Arguments"="Z= ;12.7;19.1;25.4\r", "Comments"="Anemo1", "Row No"=0, "Row Type Selector"=enum."Vertical Profile", "Completion time"="", "Row Duration (mins)"=0.0, "No. of Valid pts."=0, "Meas Setup File"="Current_Setup.xls"}, {"Start X"=-458.4, "Start Y"=87.9, "Start Z"=25.6, "End X"=-458.4, "End Y"=87.9, "End Z"=38.3, "No. of pts."=3, "Spacing"=enum."Specified", "Filename"=path "M:/\\Projects\\8773\\Results\\Tunnel1\\AnemometerSurvey.xls", "Tunnel Speed"=7.64, "Averaging time (min)"=1.0, "Extra Commands"="", "Carrier_1 Q (l/min)"=0.0, "Carrier_2 Q (l/min)"=0.0, "Trace Gas Concentration (%)"=0.0, "Specific Arguments"="Z= ;25.6;32.0;38.3\r", "Comments"="Anemo2", "Row No"=0, "Row Type Selector"=enum."Vertical Profile", "Completion time"="", "Row Duration (mins)"=0.0, "No. of Valid pts."=0, "Meas Setup File"="Current_Setup.xls"}, {"Start X"=0.0, "Start Y"=0.0, "Start Z"=150.0, "End X"=0.0, "End Y"=0.0, "End Z"=150.0, "No. of pts."=0, "Spacing"=enum."Linear", "Filename"=path "", "Tunnel Speed"=7.64, "Averaging time (min)"=0.0, "Extra Commands"="!Work in Tunnel Coordinates", "Carrier_1 Q (l/min)"=0.0, "Carrier_2 Q (l/min)"=0.0, "Trace Gas Concentration (%)"=0.0, "Specific Arguments"="", "Comments"="", "Row No"=0, "Row Type Selector"=enum."Move Traverse Only", "Completion time"="", "Row Duration (mins)"=0.0, "No. of Valid pts."=0, "Meas Setup File"=""}, {"Start X"=0.0, "Start Y"=0.0, "Start Z"=805.0, "End X"=0.0, "End Y"=0.0, "End Z"=805.0, "No. of pts."=0, "Spacing"=enum."Linear", "Filename"=path "", "Tunnel Speed"=7.64, "Averaging time (min)"=0.0, "Extra Commands"="!Work in Tunnel Coordinates", "Carrier_1 Q (l/min)"=0.0, "Carrier_2 Q (l/min)"=0.0, "Trace Gas Concentration (%)"=0.0, "Specific Arguments"="MoveTT.vi;330", "Comments"="", "Row No"=0, "Row Type Selector"=enum."Run VI Named:", "Completion time"="", "Row Duration (mins)"=0.0, "No. of Valid pts."=0, "Meas Setup File"=""}, {"Start X"=-72.9, "Start Y"=-56.5, "Start Z"=12.7, "End X"=-72.9, "End Y"=-56.5, "End Z"=25.4, "No. of pts."=3, "Spacing"=enum."Specified", "Filename"=path "M:/\\Projects\\8773\\Results\\Tunnel1\\AnemometerSurvey.xls", "Tunnel Speed"=7.64, "Averaging time (min)"=1.0, "Extra Commands"="", "Carrier_1 Q (l/min)"=0.0, "Carrier_2 Q (l/min)"=0.0, "Trace Gas Concentration (%)"=0.0, "Specific Arguments"="Z= ;12.7;19.1;25.4\r", "Comments"="Anemo1", "Row No"=0, "Row Type Selector"=enum."Vertical Profile", "Completion time"="", "Row Duration (mins)"=0.0, "No. of Valid pts."=0, "Meas Setup File"="Current_Setup.xls"}, {"Start X"=-458.4, "Start Y"=87.9, "Start Z"=25.6, "End X"=-458.4, "End Y"=87.9, "End Z"=38.3, "No. of pts."=3, "Spacing"=enum."Specified", "Filename"=path "M:/\\Projects\\8773\\Results\\Tunnel1\\AnemometerSurvey.xls", "Tunnel Speed"=7.64, "Averaging time (min)"=1.0, "Extra Commands"="", "Carrier_1 Q (l/min)"=0.0, "Carrier_2 Q (l/min)"=0.0, "Trace Gas Concentration (%)"=0.0, "Specific Arguments"="Z= ;25.6;32.0;38.3\r", "Comments"="Anemo2", "Row No"=0, "Row Type Selector"=enum."Vertical Profile", "Completion time"="", "Row Duration (mins)"=0.0, "No. of Valid pts."=0, "Meas Setup File"="Current_Setup.xls"}, {"Start X"=0.0, "Start Y"=0.0, "Start Z"=150.0, "End X"=0.0, "End Y"=0.0, "End Z"=150.0, "No. of pts."=0, "Spacing"=enum."Linear", "Filename"=path "", "Tunnel Speed"=7.64, "Averaging time (min)"=0.0, "Extra Commands"="!Work in Tunnel Coordinates", "Carrier_1 Q (l/min)"=0.0, "Carrier_2 Q (l/min)"=0.0, "Trace Gas Concentration (%)"=0.0, "Specific Arguments"="", "Comments"="", "Row No"=0, "Row Type Selector"=enum."Move Traverse Only", "Completion time"="", "Row Duration (mins)"=0.0, "No. of Valid pts."=0, "Meas Setup File"=""}, {"Start X"=0.0, "Start Y"=0.0, "Start Z"=805.0, "End X"=0.0, "End Y"=0.0, "End Z"=805.0, "No. of pts."=0, "Spacing"=enum."Linear", "Filename"=path "", "Tunnel Speed"=7.64, "Averaging time (min)"=0.0, "Extra Commands"="!Work in Tunnel Coordinates", "Carrier_1 Q (l/min)"=0.0, "Carrier_2 Q (l/min)"=0.0, "Trace Gas Concentration (%)"=0.0, "Specific Arguments"="MoveTT.vi;350", "Comments"="", "Row No"=0, "Row Type Selector"=enum."Run VI Named:", "Completion time"="", "Row Duration (mins)"=0.0, "No. of Valid pts."=0, "Meas Setup File"=""}, {"Start X"=-72.9, "Start Y"=-56.5, "Start Z"=12.7, "End X"=-72.9, "End Y"=-56.5, "End Z"=25.4, "No. of pts."=3, "Spacing"=enum."Specified", "Filename"=path "M:/\\Projects\\8773\\Results\\Tunnel1\\AnemometerSurvey.xls", "Tunnel Speed"=7.64, "Averaging time (min)"=1.0, "Extra Commands"="", "Carrier_1 Q (l/min)"=0.0, "Carrier_2 Q (l/min)"=0.0, "Trace Gas Concentration (%)"=0.0, "Specific Arguments"="Z= ;12.7;19.1;25.4\r", "Comments"="Anemo1", "Row No"=0, "Row Type Selector"=enum."Vertical Profile", "Completion time"="", "Row Duration (mins)"=0.0, "No. of Valid pts."=0, "Meas Setup File"="Current_Setup.xls"}, {"Start X"=-458.4, "Start Y"=87.9, "Start Z"=25.6, "End X"=-458.4, "End Y"=87.9, "End Z"=38.3, "No. of pts."=3, "Spacing"=enum."Specified", "Filename"=path "M:/\\Projects\\8773\\Results\\Tunnel1\\AnemometerSurvey.xls", "Tunnel Speed"=7.64, "Averaging time (min)"=1.0, "Extra Commands"="", "Carrier_1 Q (l/min)"=0.0, "Carrier_2 Q (l/min)"=0.0, "Trace Gas Concentration (%)"=0.0, "Specific Arguments"="Z= ;25.6;32.0;38.3\r", "Comments"="Anemo2", "Row No"=0, "Row Type Selector"=enum."Vertical Profile", "Completion time"="", "Row Duration (mins)"=0.0, "No. of Valid pts."=0, "Meas Setup File"="Current_Setup.xls"}, {"Start X"=0.0, "Start Y"=0.0, "Start Z"=805.0, "End X"=0.0, "End Y"=0.0, "End Z"=805.0, "No. of pts."=0, "Spacing"=enum."Linear", "Filename"=path "", "Tunnel Speed"=7.64, "Averaging time (min)"=0.0, "Extra Commands"="!Work in Tunnel Coordinates", "Carrier_1 Q (l/min)"=0.0, "Carrier_2 Q (l/min)"=0.0, "Trace Gas Concentration (%)"=0.0, "Specific Arguments"="MoveTT.vi;0.000000", "Comments"="", "Row No"=0, "Row Type Selector"=enum."Run VI Named:", "Completion time"="", "Row Duration (mins)"=0.0, "No. of Valid pts."=0, "Meas Setup File"=""}, {"Start X"=-3390.0, "Start Y"=-113.0, "Start Z"=780.0, "End X"=-3390.0, "End Y"=-113.0, "End Z"=780.0, "No. of pts."=0, "Spacing"=enum."Linear", "Filename"=path "M:/\\Projects\\8773\\Results\\Tunnel1\\AnemometerSurvey.xls", "Tunnel Speed"=0.0, "Averaging time (min)"=1.0, "Extra Commands"="!Work in Tunnel Coordinates", "Carrier_1 Q (l/min)"=0.0, "Carrier_2 Q (l/min)"=0.0, "Trace Gas Concentration (%)"=0.0, "Specific Arguments"="", "Comments"="Zeroes", "Row No"=0, "Row Type Selector"=enum."Single Measurement", "Completion time"="", "Row Duration (mins)"=0.0, "No. of Valid pts."=0, "Meas Setup File"="Current_Setup.xls"}, {"Start X"=-3390.0, "Start Y"=-113.0, "Start Z"=780.0, "End X"=-3390.0, "End Y"=-113.0, "End Z"=780.0, "No. of pts."=0, "Spacing"=enum."Linear", "Filename"=path "M:/\\Projects\\8773\\Results\\Tunnel1\\AnemometerSurvey.xls", "Tunnel Speed"=7.64, "Averaging time (min)"=1.0, "Extra Commands"="!Work in Tunnel Coordinates", "Carrier_1 Q (l/min)"=0.0, "Carrier_2 Q (l/min)"=0.0, "Trace Gas Concentration (%)"=0.0, "Specific Arguments"="", "Comments"="CalCheck", "Row No"=0, "Row Type Selector"=enum."Single Measurement", "Completion time"="", "Row Duration (mins)"=0.0, "No. of Valid pts."=0, "Meas Setup File"="Current_Setup.xls"}, {"Start X"=0.0, "Start Y"=0.0, "Start Z"=805.0, "End X"=0.0, "End Y"=0.0, "End Z"=805.0, "No. of pts."=0, "Spacing"=enum."Linear", "Filename"=path "M:/\\Projects\\8773\\Results\\Tunnel1\\AnemometerSurvey.xls", "Tunnel Speed"=7.64, "Averaging time (min)"=1.0, "Extra Commands"="!Work in Tunnel Coordinates", "Carrier_1 Q (l/min)"=0.0, "Carrier_2 Q (l/min)"=0.0, "Trace Gas Concentration (%)"=0.0, "Specific Arguments"="", "Comments"="Local CalCheck", "Row No"=0, "Row Type Selector"=enum."Single Measurement", "Completion time"="", "Row Duration (mins)"=0.0, "No. of Valid pts."=0, "Meas Setup File"="Current_Setup.xls"}, {"Start X"=-3390.0, "Start Y"=-113.0, "Start Z"=780.0, "End X"=-3390.0, "End Y"=-113.0, "End Z"=780.0, "No. of pts."=0, "Spacing"=enum."Linear", "Filename"=path "", "Tunnel Speed"=0.0, "Averaging time (min)"=0.0, "Extra Commands"="", "Carrier_1 Q (l/min)"=0.0, "Carrier_2 Q (l/min)"=0.0, "Trace Gas Concentration (%)"=0.0, "Specific Arguments"="", "Comments"="Tunnel Off", "Row No"=0, "Row Type Selector"=enum."Set Tunnel Speed Only", "Completion time"="", "Row Duration (mins)"=0.0, "No. of Valid pts."=0, "Meas Setup File"=""}] {"Carrier_2 Q (l/min)" format="%#.2f"; "Row Duration (mins)" format="%#.1f"; "Row No" min=0; "Trace Gas Concentration (%)" min=0.0 format="%#_4f"; "Carrier_1 Q (l/min)" format="%#.2f"; "Tunnel Speed" format="%#.2f"; "Start X" format="%#.2f"; "Start Y" format="%#.2f"; "Start Z" format="%#.2f"; "End X" format="%#.2f"; "End Y" format="%#.2f"; "End Z" format="%#.2f"; "Averaging time (min)" min=0.0 format="%#.2f"})   [LabVIEW 2022 SP3]
uses:
  Anemometry Sub Vis/Gen Trav/Spacing.ctl
  Anemometry Sub Vis/Controls/Multi_run_mode.ctl
  MRBRowTaskSelector.ctl
  MRCMDFBGlobal.vi
  Move Traverse Only.vi
  Set Speed Only.vi
  Single Measurement.vi
  Vertical Profile.vi
  Lateral Profile.vi
  Longitudinal Profile.vi
  Auto Calibrate.vi
  Run VI Named.vi
  MoveTTcall.vi
  TravZSurvey.vi
  Set ADAM Ch.vi
  Wait (minutes).vi
  Send Message.vi
  Blank Row.vi
panel:
  # "X           Y            Z"
  # "Start"
  # "End"
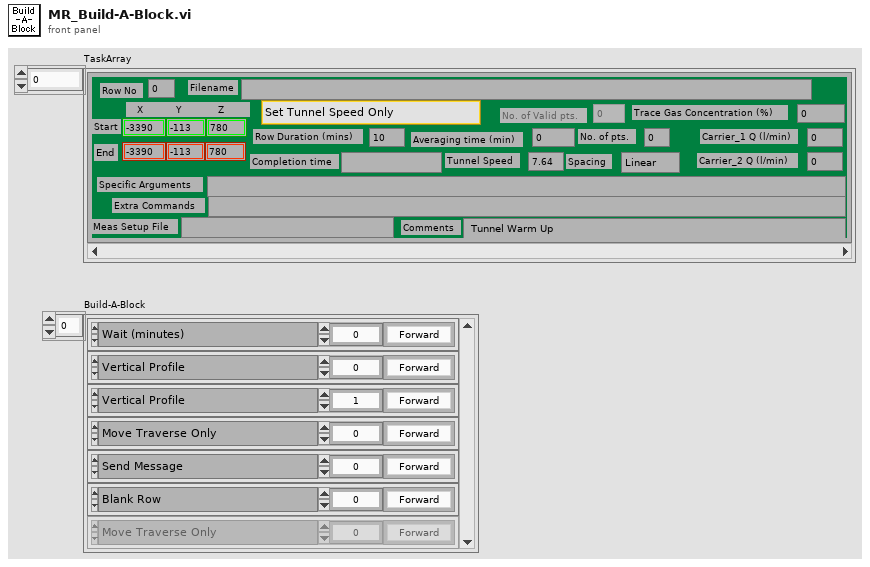
[diagram p1: front panel]
types:
  T1 = typedef "MRBRowTaskSelector.ctl" = enum16{"Move Traverse Only", "Set Tunnel Speed Only", "Set Source Only", "Set Measurement Conditions", "Single Measurement", "Vertical Profile", "Lateral Profile", "Longitudinal Profile", "Explore Volume", "Multi-Axis Profile", "Auto Calibrate", "Meas Fast FID Bkgnd", "Check Beam Power", "Scanning Valve Measurement", "Run VI Named:", "MoveTT", "TravZSurvey", "Set ADAM Ch", "Wait (minutes)", "Send Message", "Synchronize With:", "Fall Back to this Row", "Turn Off Row Repeating", "Blank Row", "Traverse 3D Volume"}
  T2 = cluster{"Row Type Selector":T1, "Index":dbl, "Direction":enum16{"Forward", "Reverse"}}[]
  T3 = typedef "Spacing.ctl" = enum16{"Linear", "Log", "Gauss", "Specified", "N/A"}
  T4 = typedef "Multi_run_mode.ctl" = enum16{"Move Traverse Only", "Set Tunnel Speed Only", "Set Source Only", "Set Measurement Conditions", "Single Measurement", "Vertical Profile", "Lateral Profile", "Longitudinal Profile", "Multi-Axis Profile", "Explore Volume", "Auto Calibrate", "Meas Fast FID Bkgnd", "Check Beam Power", "Scanning Valve Measurement", "Run VI Named:", "Set ADAM Ch", "Wait (minutes)", "Send Message", "Synchronize With:", "Fall Back to this Row", "Turn Off Row Repeating", "Traverse 3D Volume", "Blank Row", "Jump to Fall Back Row"}
  T5 = cluster{"Start X":sgl, "Start Y":sgl, "Start Z":sgl, "End X":sgl, "End Y":sgl, "End Z":sgl, "No. of pts.":i32, "Spacing":T3, "Filename":path, "Tunnel Speed":dbl, "Averaging time (min)":dbl, "Extra Commands":string, "Carrier_1 Q (l/min)":dbl, "Carrier_2 Q (l/min)":dbl, "Trace Gas Concentration (%)":dbl, "Specific Arguments":string, "Comments":string, "Row No":i32, "Row Type Selector":T4, "Completion time":string, "Row Duration (mins)":dbl, "No. of Valid pts.":i32, "Meas Setup File":string}[]
  T6 = cluster{"X":dbl, "Y":dbl, "Z":dbl, "Comment":string, "Use Tunnel Coords?":bool}[]
  T7 = cluster{"X":dbl, "Y":dbl, "Z":dbl, "Comment":string, "Use Tunnel Coords?":bool}
  T8 = typedef "RowTemplate.ctl" = cluster{"Start X":sgl, "Start Y":sgl, "Start Z":sgl, "End X":sgl, "End Y":sgl, "End Z":sgl, "No. of pts.":i32, "Spacing":T3, "Filename":path, "Tunnel Speed":dbl, "Averaging time (min)":dbl, "Extra Commands":string, "Carrier_1 Q (l/min)":dbl, "Carrier_2 Q (l/min)":dbl, "Trace Gas Concentration (%)":dbl, "Specific Arguments":string, "Comments":string, "Row No":i32, "Row Type Selector":T4, "Completion time":string, "Row Duration (mins)":dbl, "No. of Valid pts.":i32, "Meas Setup File":string}
  T9 = cluster{"Tunnel.Speed":dbl, "X":dbl, "Y":dbl, "Z":dbl, "Name":string, "Use Tunnel Coords?":bool}[]
  T10 = cluster{"Tunnel.Speed":dbl, "X":dbl, "Y":dbl, "Z":dbl, "Name":string, "Use Tunnel Coords?":bool}
  T11 = typedef "ProfCoords.ctl" = cluster{"X":dbl, "Y":dbl, "Z":dbl, "Name":string, "Spacing":enum16{"Linear", "Log", "Gauss", "Specified", "N/A"}, "start":dbl, "end":dbl, "NumPts":dbl, "Specified Locns":dbl[]}[]
  T12 = cluster{"Azimuth Array Index":u32, "Vert Prof Array Index":u32, "Lat Prof Array Index":u32, "Long Prof Array Index":u32}
  T13 = cluster{"X":dbl, "Y":dbl, "Z":dbl, "Name":string, "Spacing":enum16{"Linear", "Log", "Gauss", "Specified", "N/A"}, "start":dbl, "end":dbl, "NumPts":dbl, "Specified Locns":dbl[]}
  T14 = typedef "SingleMeas_Repeater.ctl" = cluster{"X":dbl, "Y":dbl, "Z":dbl, "Use Tunnel Coords?":bool, "RepeatEveryXDeg":dbl}
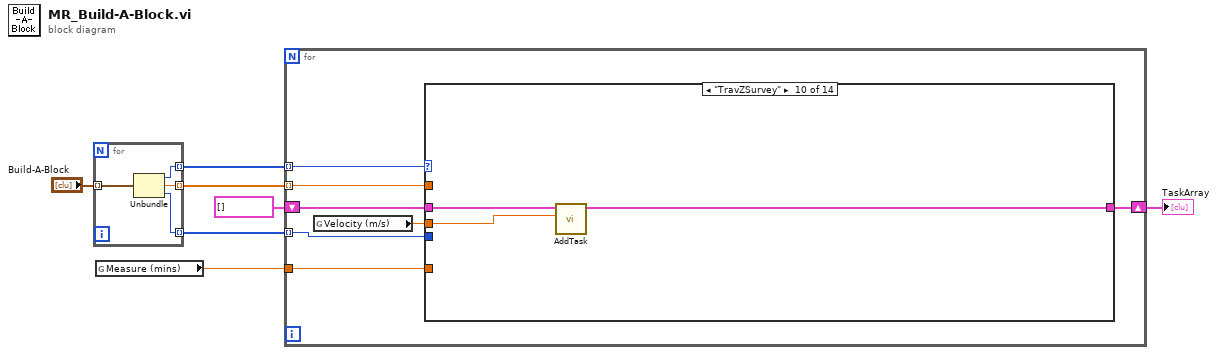
[diagram p0: block diagram]
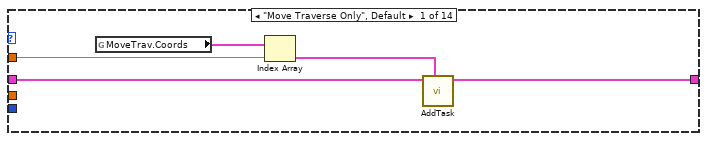
[diagram p2: hidden frame]
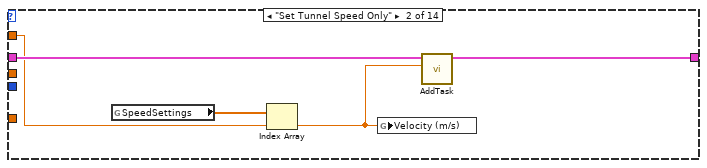
[diagram p3: hidden frame]
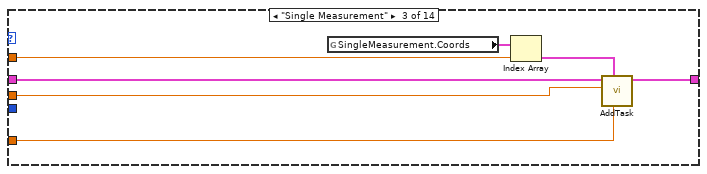
[diagram p4: hidden frame]
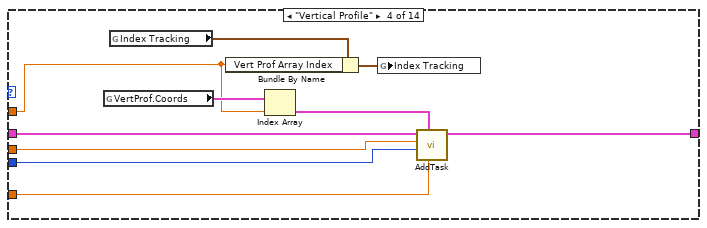
[diagram p5: hidden frame]
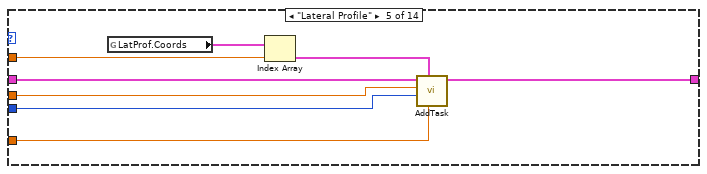
[diagram p6: hidden frame]
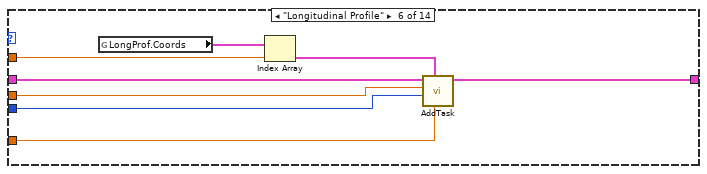
[diagram p7: hidden frame]
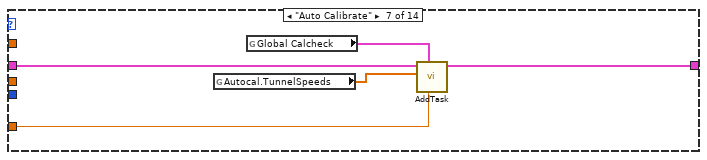
[diagram p8: hidden frame]
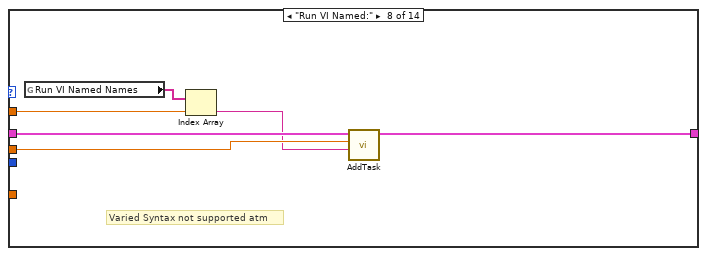
[diagram p9: hidden frame]
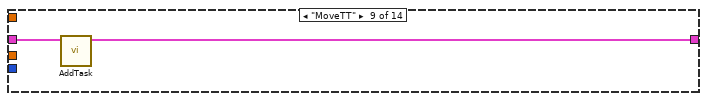
[diagram p10: hidden frame]
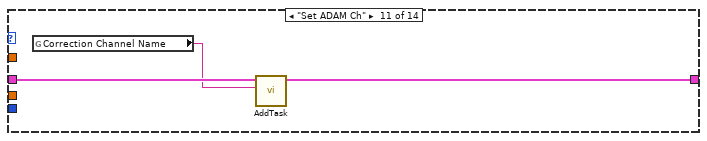
[diagram p11: hidden frame]
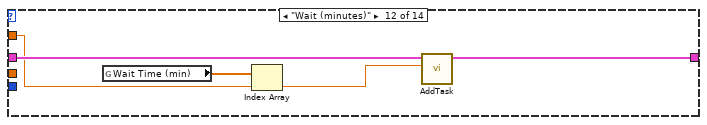
[diagram p12: hidden frame]
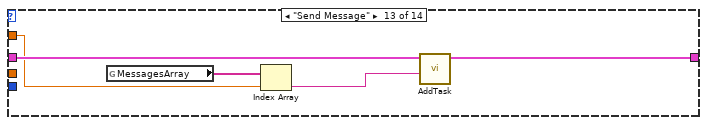
[diagram p13: hidden frame]
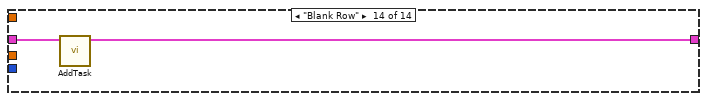
[diagram p14: hidden frame]
diagram:
  n1 = for {
    tunnel: "Build-A-Block" -> [w11] mode=indexing
    tunnel: [w10] -> w5 mode=indexing
    tunnel: [w9] -> w4 mode=indexing
    tunnel: [w8] -> w1 mode=indexing
    n2 = Unbundle(w11) -> ("Row Type Selector"=w10:T1, "Index"=w9:dbl, "Direction"=w8:enum16{"Forward", "Reverse"})
  }
  n3 = global read "MRCMDFBGlobal.vi" "Measure (mins)"() -> (w3:dbl)
  n4 = for {
    tunnel: w5 -> [w18] mode=indexing
    shift-right: [w16] -> w6
    shift-left: T5 [] -> [w17]
    tunnel: w4 -> [w15] mode=indexing
    tunnel: w3 -> [w14]
    tunnel: w1 -> [w12] mode=indexing
    n5 = global read "MRCMDFBGlobal.vi" "Velocity (m/s)"() -> (w13:dbl)
    n6 = case shown="\"TravZSurvey\"" w18 {
      tunnel: w17 -> [w23 w28 w35 w45 w53 w61 w66 w72 w74 w77 w80 w85 w90 w92]
      tunnel: [w22 w27 w34 w44 w52 w60 w65 w71 w73 w76 w79 w84 w89 w91] -> w16
      tunnel: w15 -> [w20 w26 w32 w38 w48 w56 _ w70 _ _ _ w82 w87 _]
      tunnel: w13 -> [_ _ w30 w41 w51 w59 _ w68 _ w75 _ _ _ _]
      tunnel: w14 -> [_ _ w29 w40 w50 w58 w64 _ _ _ _ _ _ _]
      tunnel: w12 -> [_ _ _ w36 w46 w54 _ _ _ _ _ _ _ _]
      frame "Move Traverse Only", Default {
        n7 = global read "MRCMDFBGlobal.vi" "MoveTrav.Coords"() -> (w21:T6)
        n8 = Index Array(array=w21, index=w20) -> (element=w19:T7)
        n9 = call-poly "AddTask.vi"("MoveTravBeforeTT 2"=w19, "Input Task Array"=w23) -> ("Output Task Array"=w22:T8[])  [unwired: 9 in]
      }
      frame "Set Tunnel Speed Only" {
        n10 = global read "MRCMDFBGlobal.vi" "SpeedSettings"() -> (w25:dbl[])
        n11 = Index Array(array=w25, index=w26) -> (element=w24:dbl)
        n12 = global write "MRCMDFBGlobal.vi" "Velocity (m/s)"(w24) -> ()
        n13 = call-poly "AddTask.vi"("Tunnel Speed"=w24, "Input Task Array"=w28) -> ("Output Task Array"=w27:T8[])  [unwired: 9 in]
      }
      frame "Single Measurement" {
        n14 = global read "MRCMDFBGlobal.vi" "SingleMeasurement.Coords"() -> (w33:T9)
        n15 = Index Array(array=w33, index=w32) -> (element=w31:T10)
        n16 = call-poly "AddTask.vi"("Averaging time (min)"=w29, "Coordinate Description"=w31, "Tunnel Speed"=w30, "Input Task Array"=w35) -> ("Output Task Array"=w34:T8[])  [unwired: 7 in]
      }
      frame "Vertical Profile" {
        n17 = global read "MRCMDFBGlobal.vi" "VertProf.Coords"() -> (w43:T11)
        n18 = global read "MRCMDFBGlobal.vi" "Index Tracking"() -> (w39:T12)
        n19 = Bundle By Name(cluster=w39, "Vert Prof Array Index"=w38) -> (w37:T12)
        n20 = Index Array(array=w43, index=w38) -> (element=w42:T13)
        n21 = global write "MRCMDFBGlobal.vi" "Index Tracking"(w37) -> ()
        n22 = call-poly "AddTask.vi"("Averaging time (min)"=w40, "Lat.Coords"=w42, "Direction"=w36, "Tunnel Speed"=w41, "Input Task Array"=w45) -> ("Output Task Array"=w44:T8[])  [unwired: 6 in]
      }
      frame "Lateral Profile" {
        n23 = global read "MRCMDFBGlobal.vi" "LatProf.Coords"() -> (w49:T11)
        n24 = Index Array(array=w49, index=w48) -> (element=w47:T13)
        n25 = call-poly "AddTask.vi"("Averaging time (min)"=w50, "Lat.Coords 2"=w47, "Direction"=w46, "Tunnel Speed"=w51, "Input Task Array"=w53) -> ("Output Task Array"=w52:T8[])  [unwired: 6 in]
      }
      frame "Longitudinal Profile" {
        n26 = global read "MRCMDFBGlobal.vi" "LongProf.Coords"() -> (w57:T11)
        n27 = Index Array(array=w57, index=w56) -> (element=w55:T13)
        n28 = call-poly "AddTask.vi"("Averaging time (min)"=w58, "Lat.Coords"=w55, "Direction"=w54, "Tunnel Speed"=w59, "Input Task Array"=w61) -> ("Output Task Array"=w60:T8[])  [unwired: 6 in]
      }
      frame "Auto Calibrate" {
        n29 = global read "MRCMDFBGlobal.vi" "Autocal.TunnelSpeeds"() -> (w62:dbl[])
        n30 = global read "MRCMDFBGlobal.vi" "Global Calcheck"() -> (w63:T14)
        n31 = call-poly "AddTask.vi"("Averaging time (min)"=w64, "Global Calcheck"=w63, "Autocal.TunnelSpeeds"=w62, "Input Task Array"=w66) -> ("Output Task Array"=w65:T8[])  [unwired: 7 in]
      }
      frame "Run VI Named:" {
        # "Varied Syntax not supported atm"
        n32 = global read "MRCMDFBGlobal.vi" "Run VI Named Names"() -> (w69:string[])
        n33 = Index Array(array=w69, index=w70) -> (element=w67:string)
        n34 = call-poly "AddTask.vi"("Specific Arguments"=w67, "Tunnel Speed"=w68, "Input Task Array"=w72) -> ("Output Task Array"=w71:T8[])  [unwired: 8 in]
      }
      frame "MoveTT" {
        n35 = call-poly "AddTask.vi"("Input Task Array"=w74) -> ("Output Task Array"=w73:T8[])  [unwired: 10 in]
      }
      frame "TravZSurvey" {
        n36 = call-poly "AddTask.vi"("Tunnel Speed"=w75, "Input Task Array"=w77) -> ("Output Task Array"=w76:T8[])  [unwired: 9 in]
      }
      frame "Set ADAM Ch" {
        n37 = global read "MRCMDFBGlobal.vi" "Correction Channel Name"() -> (w78:string)
        n38 = call-poly "AddTask.vi"("ADAM:Channel:Name"=w78, "Input Task Array"=w80) -> ("Output Task Array"=w79:T8[])  [unwired: 9 in]
      }
      frame "Wait (minutes)" {
        n39 = global read "MRCMDFBGlobal.vi" "Wait Time (min)"() -> (w83:dbl[])
        n40 = Index Array(array=w83, index=w82) -> (element=w81:dbl)
        n41 = call-poly "AddTask.vi"("Wait Time (min)"=w81, "Input Task Array"=w85) -> ("Output Task Array"=w84:T8[])  [unwired: 9 in]
      }
      frame "Send Message" {
        n42 = global read "MRCMDFBGlobal.vi" "MessagesArray"() -> (w88:string[])
        n43 = Index Array(array=w88, index=w87) -> (element=w86:string)
        n44 = call-poly "AddTask.vi"("Comments"=w86, "Input Task Array"=w90) -> ("Output Task Array"=w89:T8[])  [unwired: 9 in]
      }
      frame "Blank Row" {
        n45 = call-poly "AddTask.vi"("Input Task Array"=w92) -> ("Output Task Array"=w91:T8[])  [unwired: 10 in]
      }
    }
  }
  "TaskArray" <- w6
